vi "FRCts20_WebMethods_Comment_PUT.vi"(7 "httpRequestID":u32, 10 "comment":string, 11 "request":string) -> ()   [LabVIEW 2014, in "FRCts20_WebMethods.lvlib"]
doc: "<B>PUT</B> on the specified <B>comment</B> resource\n\n<B>Required XML Data : </B>\n<Note>\n <Solution>[<B>True</B>, <B>False</B>]</Solution>\n</Note>\n\n<B>Required HTML Post Data : </B>\nSolution: [<B>True</B>, <B>False</B>]\n\nhttp://<server address>:<port>/FRCts/request/<B>request</B>/comment/<B>comment</B>"
uses:
  FRCts20_WebMethods.lvlib
  <vilib>/wsapi/NI_WebServices.lvlib
  Backend/source/VI Source/FRCts20_Backend_API/FRCts20_Backend_API_Note.ctl
  Backend/source/VI Source/FRCts20_Backend_API/FRCts20_Backend_API_Comment.vi
  Backend/source/VI Source/FRCts20_Backend_API/FRCts20_Backend_API_Command_Note.ctl
  FRCts20_WebMethods_Redirect_Request.vi
panel:
  in  "query":string
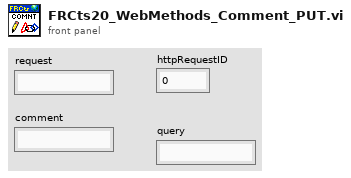
[diagram p1: front panel]
types:
  T1 = typedef "FRCts20_Backend_API.lvlib/FRCts20_Backend_API_Note.ctl" = cluster{"Note Index":u32, "Request Index":u32, "Author":string, "Time Entered":timestamp, "Text":string, "Solution":bool, "APIReturn":string}
  T2 = typedef "FRCts20_Backend_API.lvlib/FRCts20_Backend_API_Command_Note.ctl" = string
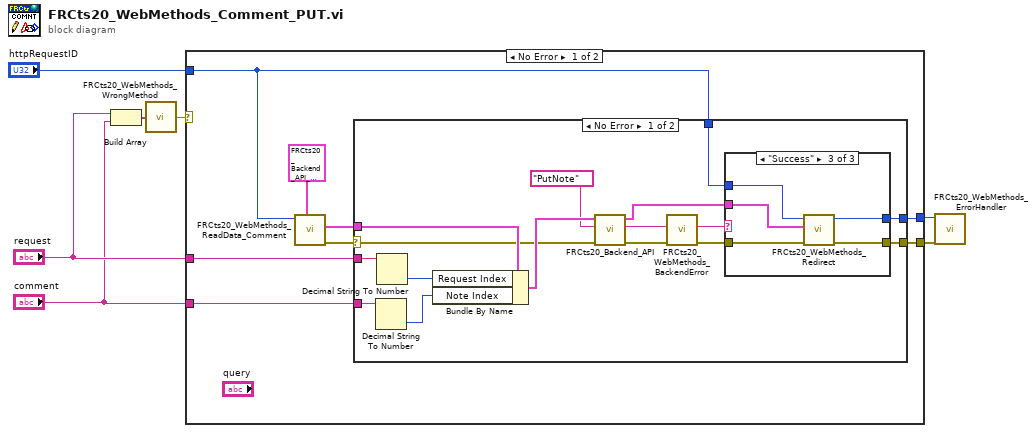
[diagram p0: block diagram]
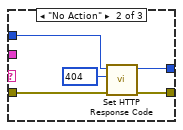
[diagram p3: hidden frame]
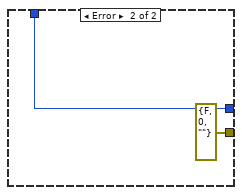
[diagram p4: hidden frame]
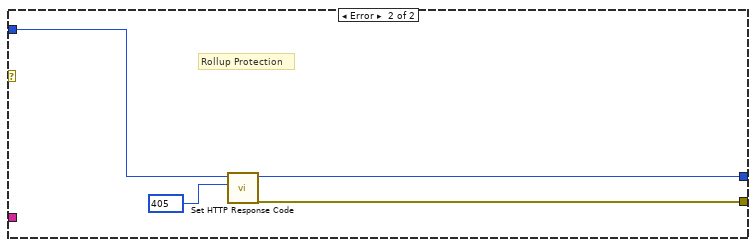
[diagram p5: hidden frame]
diagram:
  n1 = Build Array("request", "comment") -> (w6:string[])
  n2 = call "FRCts20_WebMethods_WrongMethod.vi"(4:w6) -> (1:w7)  [unwired: 3 in, 1 out]
  n3 = case shown="No Error" w7 {
    tunnel: "httpRequestID" -> [w11 w49]
    tunnel: [w10 w47] -> w3
    tunnel: [w9 w46] -> w4
    tunnel: "request" -> [w15 _]
    tunnel: "comment" -> [w14 _]
    frame No Error {
      n4 = call "FRCts20_WebMethods_ReadData_Comment.vi"("Cluster Type"=T1 {"Note Index"=0, "Request Index"=0, "Author"="", "Time Entered"=timestamp(0 s since 1904-01-01), "Text"="", "Solution"=FALSE, "APIReturn"=""} ("Note"), "httpRequestID"=w11) -> ("error out"=w8:errorcluster, "Cluster out"=w12:T1)  [unwired: 7 in, 1 out]
      n5 = case shown="No Error" w8 {
        selector: w8 -> [w16 _]
        tunnel: w15 -> [w31 _]
        tunnel: w14 -> [w30 _]
        tunnel: w12 -> [w27 _]
        tunnel: w11 -> [w20 w45]
        tunnel: [w19 w45] -> w10
        tunnel: [w18 errorcluster {"status"=FALSE, "code"=0, "source"=""} ("error out")] -> w9
        frame No Error {
          n6 = Decimal String To Number(string=w30) -> (number=w29:i32)  [unwired: 2 in, 1 out]
          n7 = Decimal String To Number(string=w31) -> (number=w28:i32)  [unwired: 2 in, 1 out]
          n8 = Bundle By Name(cluster=w27, "Request Index"=w28, "Note Index"=w29) -> (w26:T1)
          n9 = call-poly "FRCts20_Backend_API.vi"("error in (no error)"=w16, "Command"=T2 "PutNote", "Note In"=w26) -> ("error out"=w25:errorcluster, "Status"=w24:string, "Note Out"=w21:T1)  [unwired: 6 in]
          n10 = call "FRCts20_WebMethods_BackendError.vi"("error in (no error)"=w25, "Status"=w24) -> ("error out"=w23:errorcluster, "Status out"=w22:string)  [unwired: 8 in]
          n11 = case shown="\"Success\"" w22 {
            tunnel: [w33 w38 w43] -> w18
            tunnel: [w32 w37 w42] -> w19
            tunnel: w21 -> [_ _ w40]
            tunnel: w23 -> [w33 w36 w39]
            tunnel: w20 -> [w32 w35 w41]
            frame "Backend Error", Default {
            }
            frame "No Action" {
              w34 = 404 items=["100"=100, "101"=101, "200"=200, "201"=201, "202"=202, "203"=203, "204"=204, "205"=205, "206"=206, "300"=300, "301"=301, "302"=302, "303"=303, "304"=304, "305"=305, "306"=306, "307"=307, "400"=400, "401"=401, "402"=402, "403"=403, "404"=404, "405"=405, "406"=406, "407"=407, "408"=408, "409"=409, "410"=410, "411"=411, "412"=412, "413"=413, "414"=414, "415"=415, "416"=416, "417"=417, "500"=500, "501"=501, "502"=502, "503"=503, "504"=504, "505"=505] ("response code (200)")
              n12 = call <vilib>:"Set HTTP Response Code.vi"("error in (no error)"=w36, "response code (200)"=w34, "httpRequestID"=w35) -> ("error out"=w38:errorcluster, "httpRequestID out"=w37:u32)  [unwired: 7 in]
            }
            frame "Success" {
              n13 = call-poly "FRCts20_WebMethods_Redirect.vi"("error in (no error)"=w39, "Request"=w40, "httpRequestID"=w41) -> ("error out"=w43:errorcluster, "httpRequestID out"=w42:u32)  [unwired: 7 in]
            }
          }
        }
        frame Error {
        }
      }
    }
    frame Error {
      w48 = 405 items=["100"=100, "101"=101, "200"=200, "201"=201, "202"=202, "203"=203, "204"=204, "205"=205, "206"=206, "300"=300, "301"=301, "302"=302, "303"=303, "304"=304, "305"=305, "306"=306, "307"=307, "400"=400, "401"=401, "402"=402, "403"=403, "404"=404, "405"=405, "406"=406, "407"=407, "408"=408, "409"=409, "410"=410, "411"=411, "412"=412, "413"=413, "414"=414, "415"=415, "416"=416, "417"=417, "500"=500, "501"=501, "502"=502, "503"=503, "504"=504, "505"=505] ("response code (200)")
      # "Rollup Protection"
      n14 = call <vilib>:"Set HTTP Response Code.vi"("response code (200)"=w48, "httpRequestID"=w49) -> ("error out"=w46:errorcluster, "httpRequestID out"=w47:u32)  [unwired: 8 in]
    }
  }
  n15 = call "FRCts20_WebMethods_ErrorHandler.vi"("error in"=w4, "LabVIEW Web Service Request"=w3) -> ()  [unwired: 8 in, 2 out]
